vi "Instance RepCap.vi"(0 "Instance In":T1=1, 1 "RepCap String In (\"\")":string) -> (2 "In Range?":bool, 3 "RepCap Identifier Out":string)   [LabVIEW 2020, in "Rohde&Schwarz CMWXP NR FR1 Measurement.lvlib"]
doc: "Selects the Instance repeated capability identifier for the selected Instance value, and optionally appends it to the end of the repeated capability identifier string wired in to the RepCap String In terminal. The output string can be wired into the Repeated Capabilities terminal of the rscmxpnrfr2m ExpressVI."
uses:
  <instrlib>/Rohde&Schwarz CMWXP NR FR1 Measurement/Rohde&Schwarz CMWXP NR FR1 Measurement.lvlib
  <instrlib>/Rohde&Schwarz CMWXP NR FR1 Measurement/Private/_Instance.ctl
  <instrlib>/Rohde&Schwarz CMWXP NR FR1 Measurement/Public/Utility/rsidr_core_global.vi
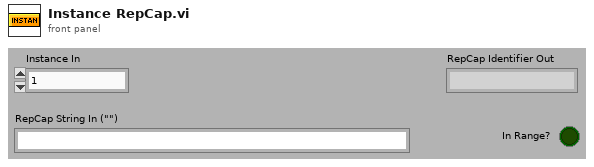
[diagram p1: front panel]
types:
  T1 = typedef "Rohde&Schwarz CMWXP NR FR1 Measurement.lvlib/_Instance.ctl" = i32
  T2 = cluster{"repCapName":string, "identifiers":string[], "cmdValues":string[]}[]
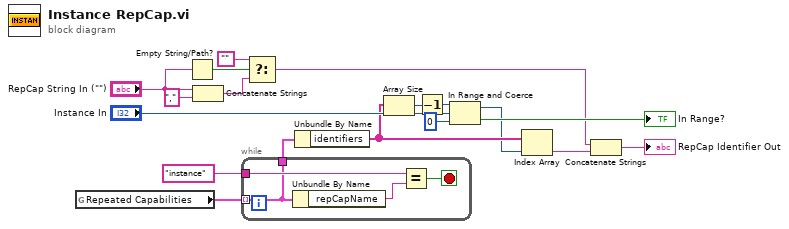
[diagram p0: block diagram]
diagram:
  n1 = global read "rsidr_core_global.vi" "Repeated Capabilities"() -> (w3:T2)
  n2 = Empty String/Path?(string/path="RepCap String In (\"\")") -> (empty?=w5:bool)
  n3 = Concatenate Strings("RepCap String In (\"\")", "," ("string")) -> (w8:string)
  n4 = while {
    tunnel: "instance" -> [w21]
    tunnel: w3 -> [w19] mode=indexing
    tunnel: [w19] -> w12
    stop <- w20 stop-if-true
    n5 = Unbundle By Name(w19) -> ("repCapName"=w22:string)
    n6 = Equal?(x=w21, y=w22) -> (x = y?=w20:bool)
  }
  n7 = Select(t="" ("Empty String Constant"), s=w5, f=w8) -> (s? t:f=w6:string)
  n8 = Unbundle By Name(w12) -> ("identifiers"=w16:string[])
  n9 = Array Size(array=w16) -> (size(s)=w15:i32)
  n10 = Decrement(x=w15) -> (x-1=w2:i32)
  n11 = In Range and Coerce(upper limit=w2, x="Instance In", lower limit=0) -> (coerced(x)=w1:T1, In Range?=→"In Range?":bool)
  n12 = Index Array(array=w16, index=w1) -> (element=w10:string)
  n13 = Concatenate Strings(w6, w10) -> (→"RepCap Identifier Out":string)
